vi "RescaleGraphs.vi"(0 "WaveformGraph in":refnum<vi>, 1 "Offset (V) 3":dbl, 2 "Range (V) 3":dbl, 3 "Preliminary Histogram":refnum<vi>) -> ()   [LabVIEW 2012]
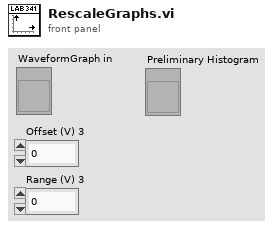
[diagram p1: front panel]
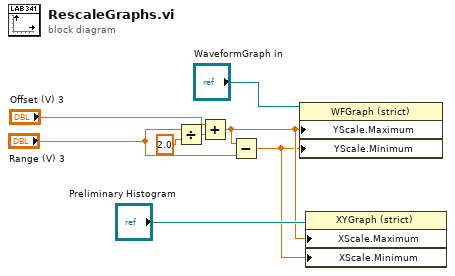
[diagram p0: block diagram]
diagram:
  n1 = Divide(x="Range (V) 3", y=2.0) -> (x/y=w5:dbl)
  n2 = Add(x="Offset (V) 3", y=w5) -> (x+y=w2:dbl)
  n3 = Subtract(x=w2, y="Range (V) 3") -> (x-y=w1:dbl)
  n4 = property on="Property Node" class="WFGraph (strict)"(reference="WaveformGraph in", "YScale.Maximum"=w2, "YScale.Minimum"=w1) -> ()  [unwired: 1 in, 2 out]
  n5 = property on="Property Node" class="XYGraph (strict)"(reference="Preliminary Histogram", "XScale.Maximum"=w2, "XScale.Minimum"=w1) -> ()  [unwired: 1 in, 2 out]
